vi "SubVI_ReleaseSingle.vi"(8 "error in (no error)":errorcluster, 11 "Handle":u32) -> (0 "error out":errorcluster)   [LabVIEW 2023, in "ADS_Library.lvlib"]
uses:
  ADS_Library.lvlib
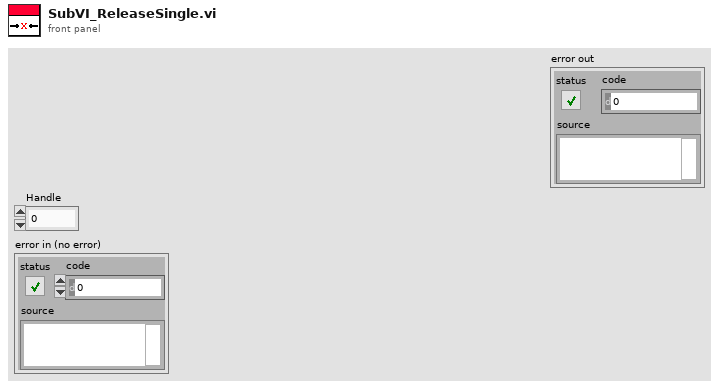
[diagram p1: front panel]
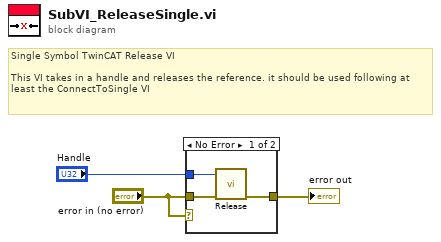
[diagram p0: block diagram]
diagram:
  # "Single Symbol TwinCAT Release VI\n\nThis VI takes in a handle and releases the reference. it should be used following at least the ConnectToSingle VI"
  n1 = case shown="No Error" "error in (no error)" {
    tunnel: [w6 w7] -> w3
    tunnel: "Handle" -> [w5 _]
    tunnel: "error in (no error)" -> [w4 w7]
    frame No Error {
      n2 = call <userlib>:"Release.vi"("Handle"=w5, "error in (no error)"=w4) -> ("error out"=w6:errorcluster)  [unwired: 13 in]
    }
    frame Error {
    }
  }
  "error out" <- w3
